vi "Configure Measurement (Reflection Measurement).vi"(0 "VISA resource name":refnum<visa-resource-name>, 1 "Enable IIM (F: Disable)":bool, 5 "Measurement Type (0: Reflection)":i32(ring) items=["Reflection", "One Port Insertion Loss", "Distance to Fault"], 9 "Calibration Type (0: Selected)":i32(ring) items=["Selected", "Full"], 11 "error in (no error)":errorcluster) -> (4 "VISA resource name out":refnum<visa-resource-name>, 15 "error out":errorcluster)   [LabVIEW 2022 SP3, in "Agilent N934X Series.lvlib"]
doc: "Configures the general setting of Reflection Measurement Option.\n\nNotes:\n(1) Option RM7 and TG7 are required to enable the reflection measurement function.\n\n(2) This VI is only applicable for N9321C, N9322C, N9323C, N9324C models."
uses:
  <instrlib>/Agilent N934X Series/Agilent N934X Series.lvlib
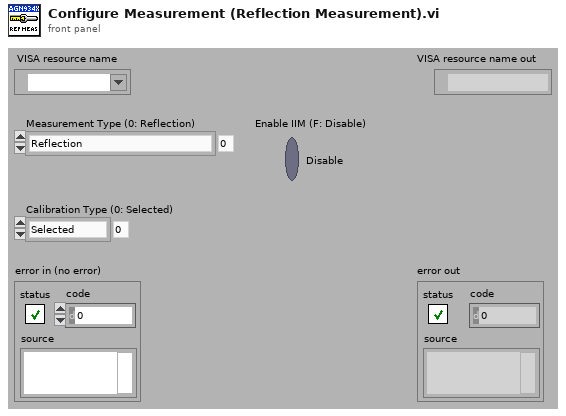
[diagram p1: front panel]
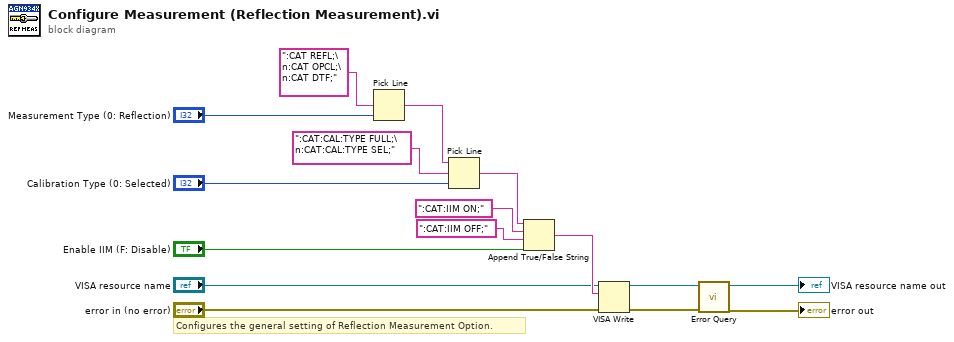
[diagram p0: block diagram]
diagram:
  # "Configures the general setting of Reflection Measurement Option."
  n1 = Pick Line(multi-line string=":CAT REFL;\n:CAT OPCL;\n:CAT DTF;", line index="Measurement Type (0: Reflection)") -> (output string=w12:string)  [unwired: 1 in]
  n2 = Pick Line(string ("")=w12, multi-line string=":CAT:CAL:TYPE FULL;\n:CAT:CAL:TYPE SEL;", line index="Calibration Type (0: Selected)") -> (output string=w11:string)
  n3 = Append True/False String(1:"Enable IIM (F: Disable)", 2:":CAT:IIM OFF;", 3:":CAT:IIM ON;", 4:w11) -> (0:w7:string)
  n4 = VISA Write(VISA resource name="VISA resource name", write buffer=w7, error in (no error)="error in (no error)") -> (VISA resource name out=w4:refnum<visa-resource-name>, error out=w3:errorcluster)  [unwired: 1 out]
  n5 = call <instrlib>:"Error Query.vi"("error in (no error)"=w3, "VISA resource name"=w4) -> ("error out"=→"error out":errorcluster, "VISA resource name out"=→"VISA resource name out":refnum<visa-resource-name>)  [unwired: 6 in, 2 out]
